vi "LiftControl.vi"(1 "Y-axis Value":dbl) -> ()   [LabVIEW 2014]
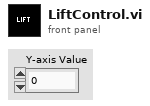
[diagram p1: front panel]
types:
  T1 = typedef "WPI_SwitchDevRef.ctl" = cluster{"DevStatus":errorcluster, "DIO Channel":T2, "Controller":T3, "CntIndex":T4, "Normally Closed":bool}
  T2 = typedef "FPGA_DIOChannel.ctl" = enum8{"DIO 0", "DIO 1", "DIO 2", "DIO 3", "DIO 4", "DIO 5", "DIO 6", "DIO 7", "DIO 8", "DIO 9", "DIO MXP 0", "DIO MXP 1", "DIO MXP 2", "DIO MXP 3", "DIO MXP 4", "DIO MXP 5", "DIO MXP 6", "DIO MXP 7", "DIO MXP 8", "DIO MXP 9", "DIO MXP 10", "DIO MXP 11", "DIO MXP 12", "DIO MXP 13", "DIO MXP 14", "DIO MXP 15", "Invalid"}
  T3 = typedef "FPGA_TypedefDigitalModule.ctl" = enum16{"Controller 1"}
  T4 = typedef "FPGA_CounterCtrSystemIndex.ctl" = enum8{"Ctr 0", "Ctr 1", "Ctr 2", "Ctr 3", "Ctr 4", "Ctr 5", "Ctr 6", "Ctr 7", "Invalid"}
  T5 = typedef "WPI_MotorControlDeviceRef.ctl" = cluster{"DeviceStatus":errorcluster, "Type":T6, "PWM":cluster{"Controller":T3, "PWM Channel":T7, "DeadBand":T8}, "CAN":cluster{"Device Number":u8, "Control Mode":T9, "Semaphore":T10, "Max Vout":dbl, "TalonSRX Control Mode":T11}, "Invert":bool, "TransformRef":T12, "InvTransformRef":T12}
  T6 = typedef "WPI_MotorControlType.ctl" = enum16{"PWM", "CAN", "CANTalonSRX"}
  T7 = typedef "FPGA_DIOPWMChannel.ctl" = enum8{"PWM 0", "PWM 1", "PWM 2", "PWM 3", "PWM 4", "PWM 5", "PWM 6", "PWM 7", "PWM 8", "PWM 9", "PWM MXP 0", "PWM MXP 1", "PWM MXP 2", "PWM MXP 3", "PWM MXP 4", "PWM MXP 5", "PWM MXP 6", "PWM MXP 7", "PWM MXP 8", "PWM MXP 9", "Invalid"}
  T8 = typedef "WPI_PWMDeadband.ctl" = cluster{"Name":string, "maxPositivePwm":i32, "minPositivePwm":i32, "centerPwm":i32, "maxNegativePwm":i32, "minNegativePwm":i32, "angularRange":u16}
  T9 = typedef "WPI_CANJaguar_ControlMode.ctl" = enum8{"Percent VBus", "Current", "Speed", "Position", "Voltage"}
  T10 = typedef "Semaphore RefNum" = refnum<k1>
  T11 = typedef "WPI_CANTalonSRX_APIControlMode.ctl" = enum8{"Percent VBus", "Speed", "Position", "Slave", "Unchanged / Invalid"}
  T12 = typedef "WPI_PWMTransform_ConPane.ctl" = refnum<vi>
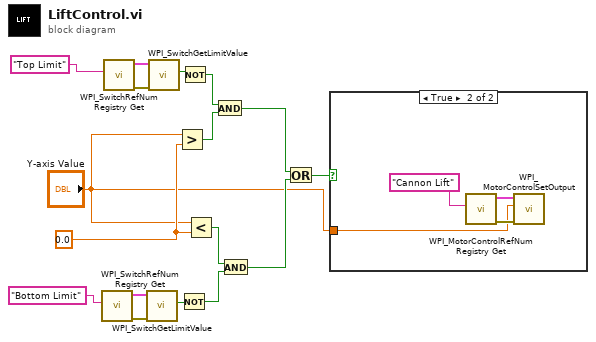
[diagram p0: block diagram]
diagram:
  w17 = 0.0
  n1 = call <vilib>:"WPI_SwitchRefNum Registry Get.vi"("refnum name"="Bottom Limit") -> ("error out"=w13:errorcluster, "SwitchDevRef"=w12:T1)  [unwired: 9 in]
  n2 = call <vilib>:"WPI_SwitchRefNum Registry Get.vi"("refnum name"="Top Limit") -> ("error out"=w16:errorcluster, "SwitchDevRef"=w15:T1)  [unwired: 9 in]
  n3 = call <vilib>:"WPI_SwitchGetLimitValue.vi"("error in (no error)"=w13, "SwitchDevRef"=w12) -> ("Switch Pressed"=w9:bool)  [unwired: 7 in, 2 out]
  n4 = call <vilib>:"WPI_SwitchGetLimitValue.vi"("error in (no error)"=w16, "SwitchDevRef"=w15) -> ("Switch Pressed"=w10:bool)  [unwired: 7 in, 2 out]
  n5 = Greater?(x="Y-axis Value", y=w17) -> (0:w5:bool)
  n6 = Not(x=w9) -> (.not. x?=w7:bool)
  n7 = Not(x=w10) -> (.not. x?=w6:bool)
  n8 = Less?(x="Y-axis Value", y=w17) -> (x < y?=w8:bool)
  n9 = And(x=w6, y=w5) -> (x .and. y?=w3:bool)
  n10 = And(x=w8, y=w7) -> (x .and. y?=w2:bool)
  n11 = Or(x=w3, y=w2) -> (x .or. y?=w4:bool)
  n12 = case shown="True" w4 {
    tunnel: "Y-axis Value" -> [_ w18]
    frame False {
    }
    frame True {
      n13 = call <vilib>:"WPI_MotorControlRefNum Registry Get.vi"("refnum name"="Cannon Lift") -> ("error out"=w20:errorcluster, "MotorControlDevRef"=w19:T5)  [unwired: 9 in]
      n14 = call <vilib>:"WPI_MotorControlSetOutput.vi"("error in (no error)"=w20, "Output"=w18, "MotorControlDevRef"=w19) -> ()  [unwired: 6 in, 3 out]
    }
  }
